vi "test Deployment No Configuration.vi"(8 "error in (no error)":errorcluster, 11 "TestCase in":refnum<class "Deployment.lvclass">) -> (0 "error out":errorcluster, 3 "TestCase out":refnum<class "Deployment.lvclass">)   [LabVIEW 2020, in "Deployment.lvclass"]
uses:
  Deployment.lvclass
  <vilib>/addons/_JKI Toolkits/VI Tester/TestCase.llb/TestCase.lvclass
  315b1c3a-44c8-49e8-b756-01f865c29b4a.vi
  C:/git/ni/niveristand-custom-device-testing-tools/VeriStandTestCase/VeriStandTestCase.lvclass
  C:/Program Files (x86)/National Instruments/LabVIEW 2020/vi.lib/addons/_JKI Toolkits/VI Tester/TestCase.llb/TestCase.lvclass
  C:/git/ni/niveristand-ballard-milStd1553-custom-device/Source/Custom Device Support/Tests/System/Deployment/Deployment.lvclass
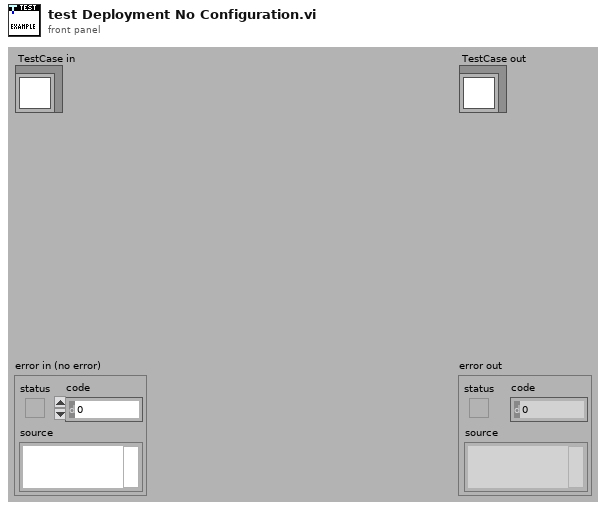
[diagram p1: front panel]
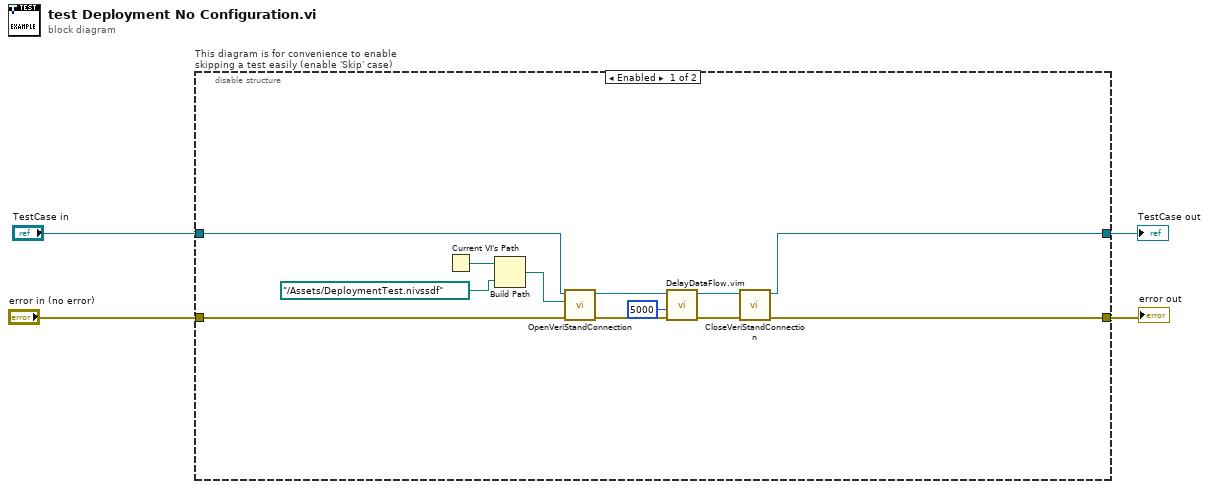
[diagram p0: block diagram]
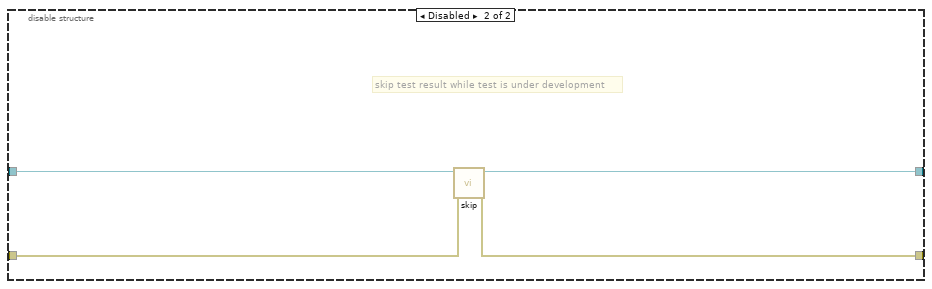
[diagram p2: hidden frame]
diagram:
  n1 = disable-structure "This diagram is for convenience to enable skipping a test easily (enable 'Skip' case)" shown="Enabled" {
    disable-tunnel: "TestCase in" -> [w11 w19]
    disable-tunnel: [w5 w17] -> w1
    disable-tunnel: [w7 w18] -> w3
    disable-tunnel: "error in (no error)" -> [w12 w16]
    frame Enabled {
      n2 = Current VI's Path() -> (path=w15:path)
      n3 = Build Path(base path=w15, name or relative path=path "../Assets/DeploymentTest.nivssdf" ("Hardware File Path")) -> (appended path=w13:path)
      n4 = call-dynamic "OpenVeriStandConnection.vi"("error in (no error)"=w12, "System Definition File"=w13, "VeriStand Test Case in"=w11) -> ("error out"=w10:errorcluster, "VeriStand Test Case out"=w6:refnum<class "Deployment.lvclass">)  [unwired: 6 in, 1 out]
      n5 = call "DelayDataFlow.vim"("value in"=w10, "milliseconds to wait"=u32 5000) -> ("value out"=w8:errorcluster)  [unwired: 2 in, 1 out]
      n6 = call-dynamic "CloseVeriStandConnection.vi"("error in (no error)"=w8, "VeriStand Test Case in"=w6) -> ("error out"=w7:errorcluster, "VeriStand Test Case out"=w5:refnum<class "Deployment.lvclass">)  [unwired: 8 in]
    }
    frame Disabled {
      # "skip test result while test is under development"
      n7 = call <vilib>:"skip.vi"("error in (no error)"=w16, "TestCase in"=w19) -> ("error out"=w18:errorcluster, "TestCase out"=w17:refnum<class "Deployment.lvclass">)  [unwired: 8 in]
    }
  }
  "error out" <- w3
  "TestCase out" <- w1
